vi "basement tank 4.vi"() -> ()   [LabVIEW 2019]
uses:
  <vilib>/NI/Current Value Table/Type Defs/Single Tag.ctl
  <vilib>/NI/Current Value Table/Type Defs/Data Types.ctl
  <vilib>/NI/STM/TCP/Read Meta Data (TCP Ref).vi
  <vilib>/NI/STM/TCP/Get Connection Reference (TCP).vi
  <vilib>/NI/AMC/Read Termination Message.vi
  <vilib>/NI/AMC/Create Single Message.vi
  <vilib>/NI/AMC/Update Message Routing Info.vi
  <vilib>/NI/STM/TCP/Read Meta Data (TCP Clst).vi
  <vilib>/NI/AMC/Globals.vi
  <vilib>/NI/STM/TCP/Write Message (TCP).vi
  <vilib>/NI/AMC/Send Message.vi
  <vilib>/NI/AMC/AMC.lvlib
  <vilib>/NI/STM/NI STM.lvlib
  <vilib>/NI/Current Value Table/Current Value Table.lvlib
panel:
  in  "Specific Gravity":dbl(knob)=1.0 min=1.0 max=1.25 step=0.0025 scale=1.0..1.25
  in  "Pump Speed (%)":dbl(knob) scale=10.0..100.0
  out "Boiler Water Out":dbl(knob) scale=10.0..110.0
  out "Boiler Water In":dbl(knob) scale=10.0..110.0
  out "Tempered Water Out":dbl(knob) scale=10.0..35.0
  out "Tempered Water In":dbl(knob) scale=10.0..35.0
  out "Chilled Water Out":dbl(knob) scale=0.0..25.0
  out "Chilled Water In":dbl(knob) scale=0.0..25.0
  in  "Tab Control":enum32{"Main Pump"}(tab)
  out "Amps":dbl format="%#.2g"
  out "Volts":dbl format="%#.1f"
  out "VFD T":dbl format="%#.2g"
  out "RPM":dbl format="%#.2f"
  out "Fault Code":dbl format="%#.2g"
  out "Freq":dbl format="%#.2g"
  out "Main Pump":bool
  out "Total Added":dbl format="%.2g"
  out "DI Flow (L/min)":dbl(knob) scale=0.0..100.0
  in  "Liters DI to Add":dbl(knob) min=0.0 max=500.0 step=1.0 scale=0.0..500.0
  in  "Add DI Water":bool
  in  "Drain System to Tree":bool
  in  "Enable Main Pump":bool
  out "E Stop":bool
  out "Run Enabled?":bool
  out "Tank":dbl(slide) scale=0.0..1500.0
  in  "Machine":bool
  in  "Basement 4":bool
  in  "Dryer":bool
  in  "Rinse 4":bool
  in  "Rinse 3":bool
  in  "Rinse 2":bool
  in  "Basement 3":bool
  in  "Basement 2":bool
  in  "Basement 1":bool
  in  "Plater 6":bool
  in  "Plater 5":bool
  in  "Plater 4":bool
  in  "Plater 3":bool
  in  "Plater 2":bool
  in  "Plater 1":bool
  in  "Predip":bool
  in  "Rinse 1":bool
  in  "Cleaner":bool
  in  "Etch":bool
  out "status":string
  out "Tnk1Tee":bool
  out "PipeToPump":bool
  # "Module Selection"
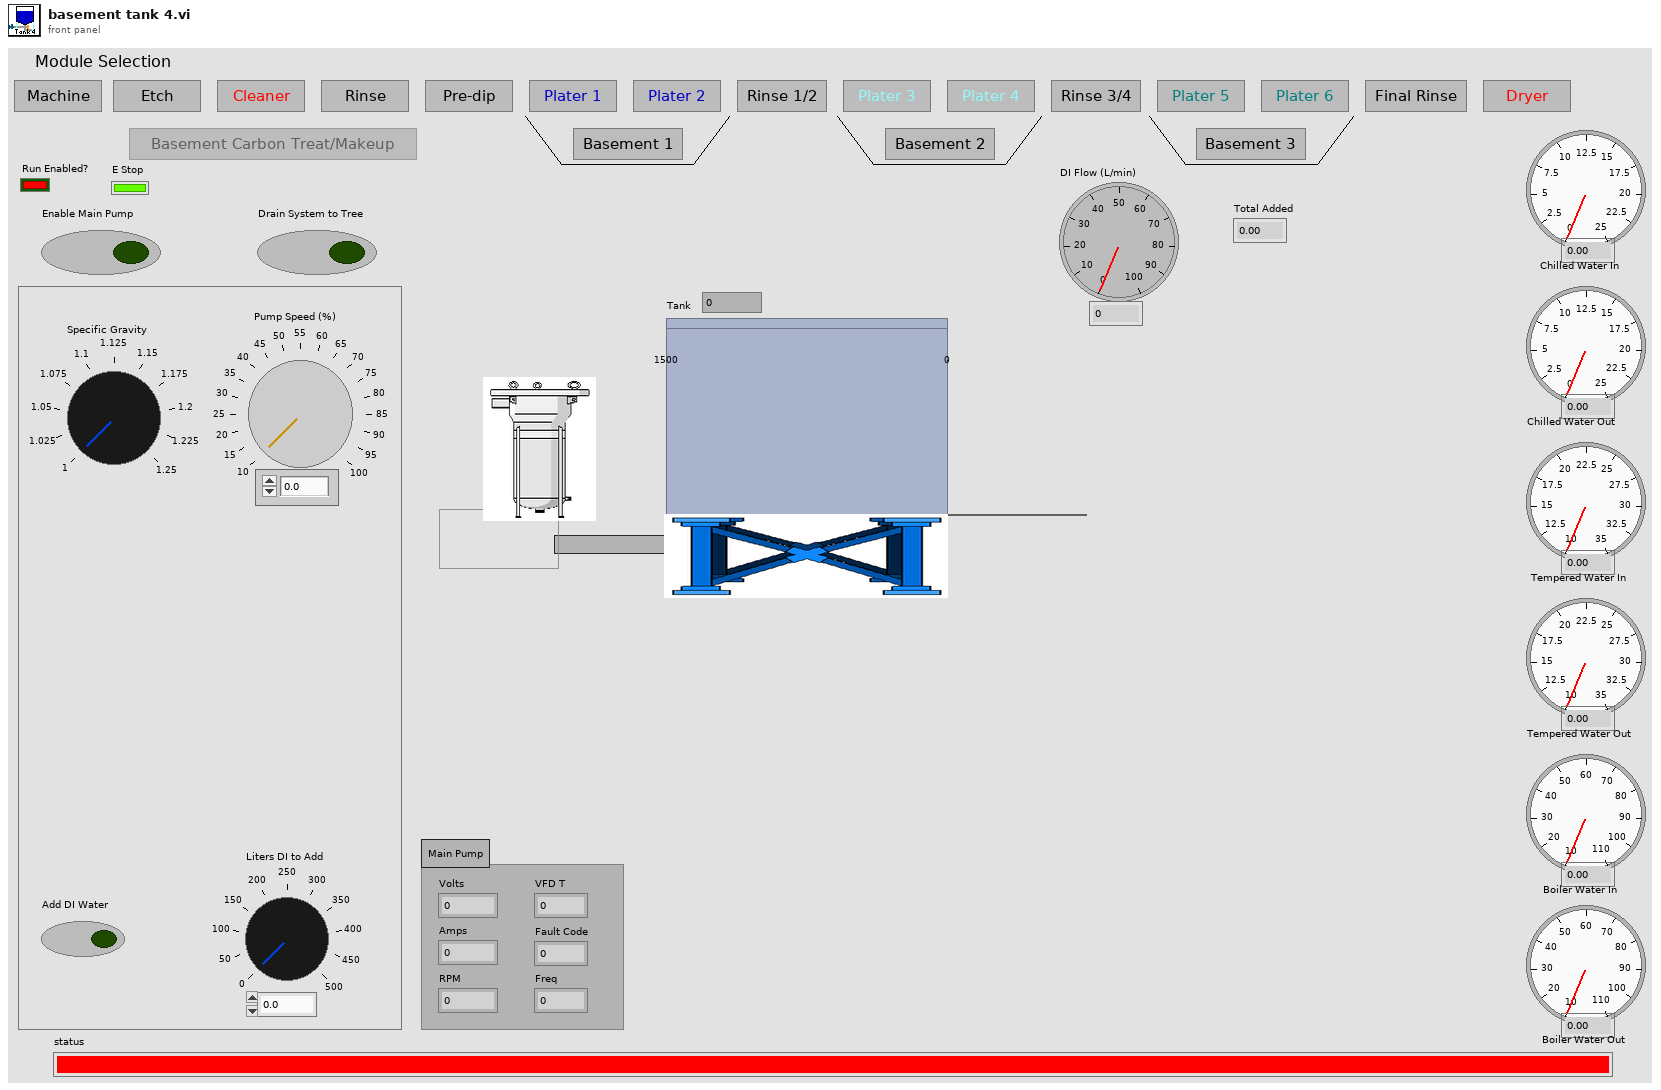
[diagram p1: front panel]
types:
  T1 = typedef "Current Value Table.lvlib/Single Tag.ctl" = cluster{"Data Type":T2, "Name":string, "Value":string, "Description":string}
  T2 = typedef "Current Value Table.lvlib/Data Types.ctl" = enum16{"Double", "Single", "I64", "I32", "I16", "I8", "U64", "U32", "U16", "U8", "String", "Boolean", "Array of U8", "Array of U16", "Array of U32", "Array of U64", "Array of I64", "Array of I32", "Array of I16", "Array of I8", "Array of Double", "Array of Single", "Array of Boolean", "Array of String"}
  T3 = typedef "NI STM.lvlib/TCP Connection Info.ctl" = cluster{"connection ID":refnum<k5>, "meta data":T4[]}
  T4 = typedef "NI STM.lvlib/MetaDataElement.ctl" = string
  T5 = typedef "AMC.lvlib/Message Queue.ctl" = refnum<queue>
  T6 = enum8{"Enabled", "Disabled", "Disabled and Grayed Out"}
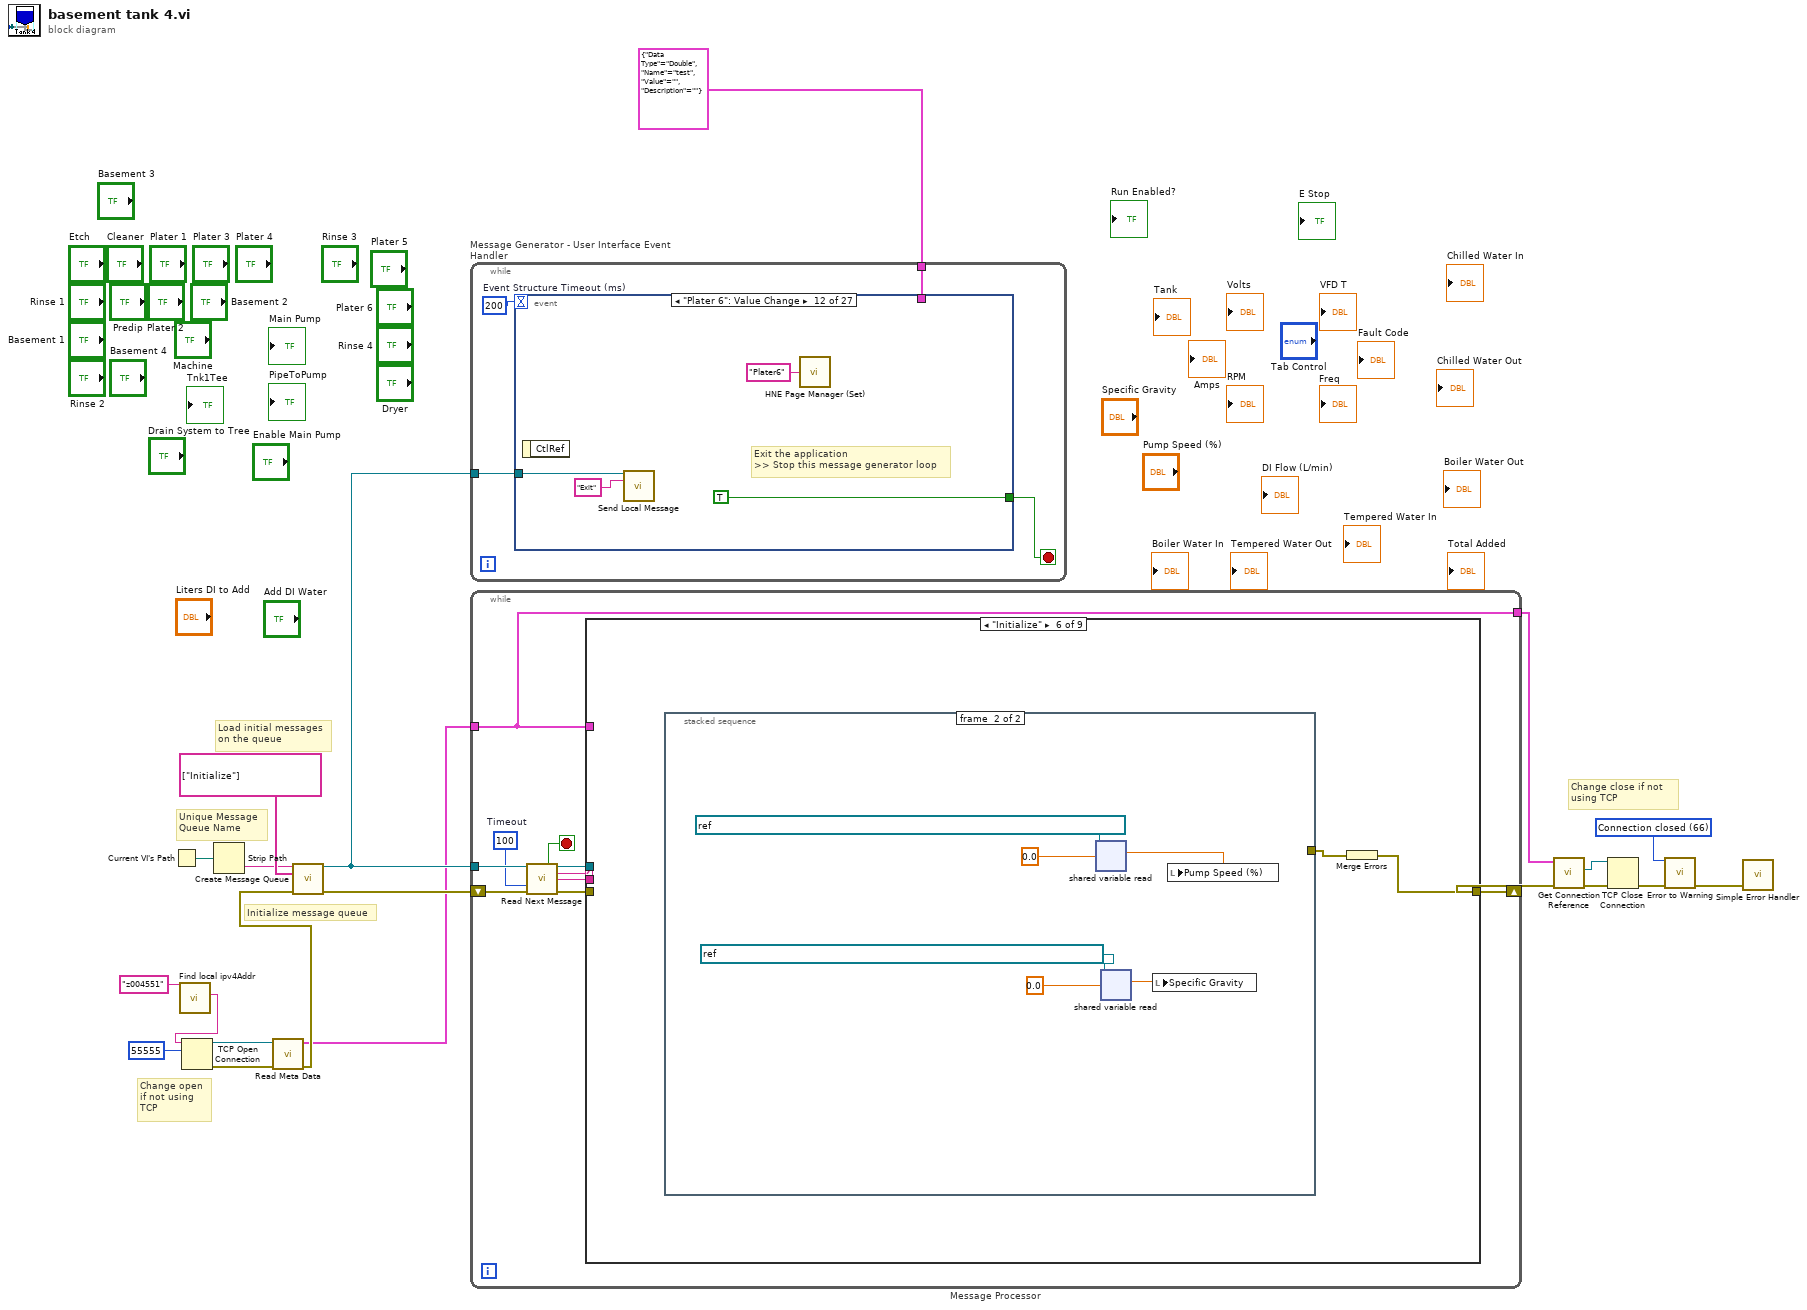
[diagram p0: block diagram]
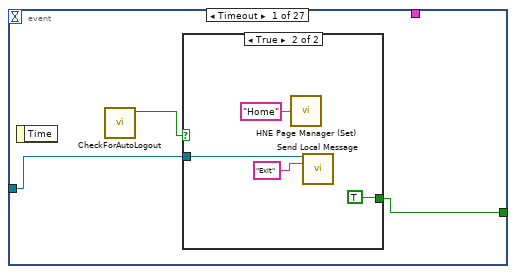
[diagram p2: hidden frame]
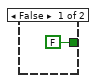
[diagram p3: hidden frame]
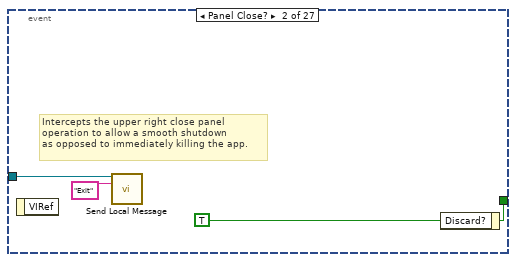
[diagram p4: hidden frame]
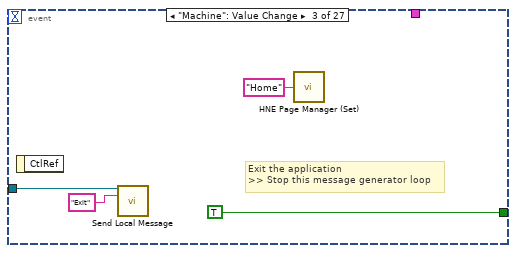
[diagram p5: hidden frame]
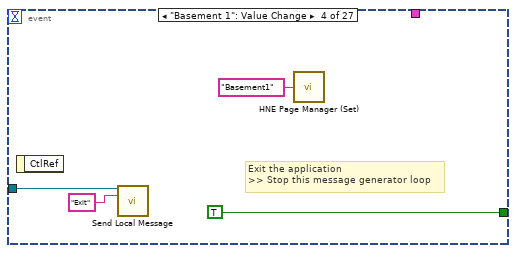
[diagram p6: hidden frame]
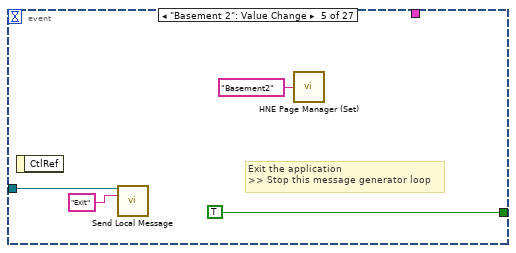
[diagram p7: hidden frame]
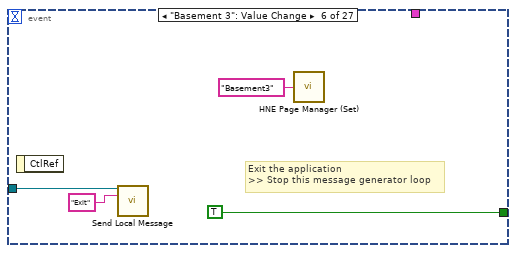
[diagram p8: hidden frame]
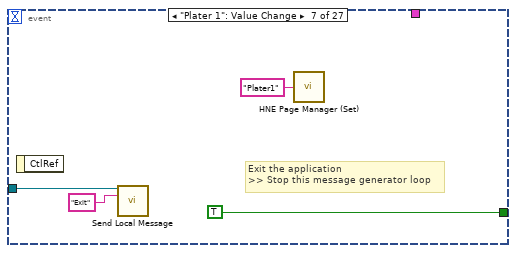
[diagram p9: hidden frame]
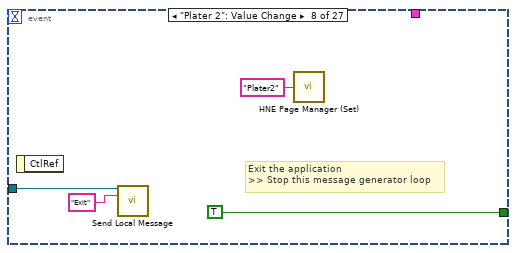
[diagram p10: hidden frame]
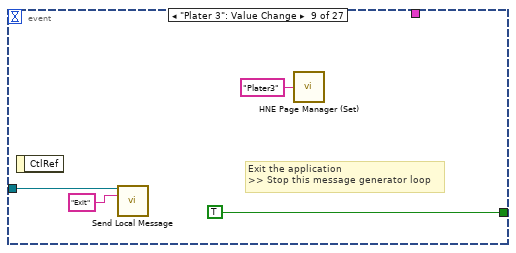
[diagram p11: hidden frame]
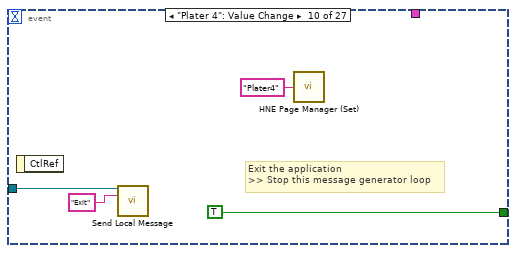
[diagram p12: hidden frame]
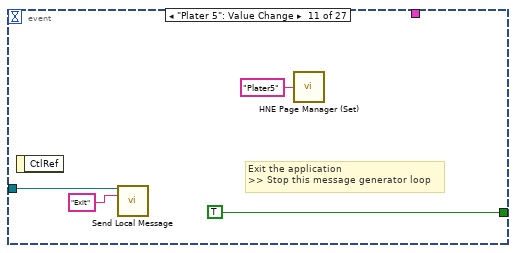
[diagram p13: hidden frame]
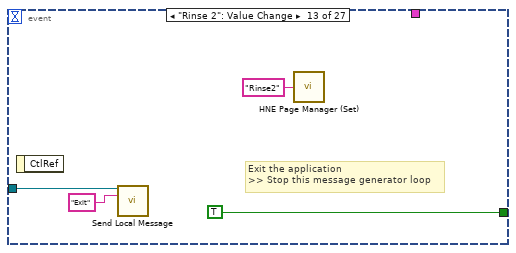
[diagram p14: hidden frame]
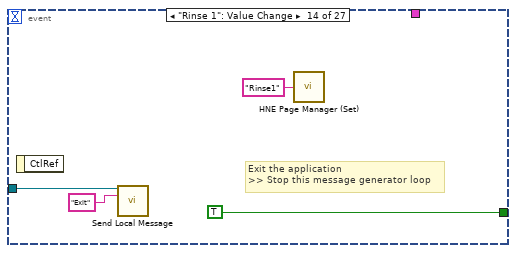
[diagram p15: hidden frame]
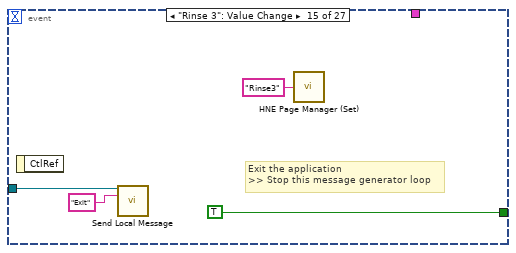
[diagram p16: hidden frame]
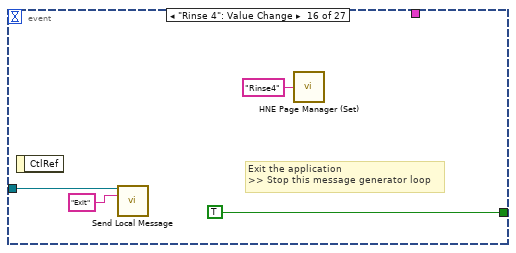
[diagram p17: hidden frame]
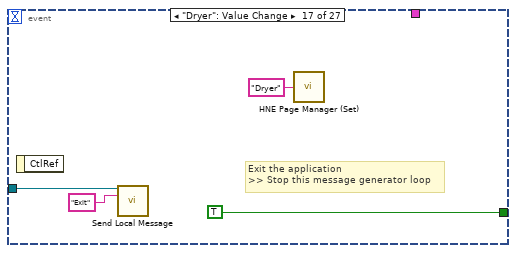
[diagram p18: hidden frame]
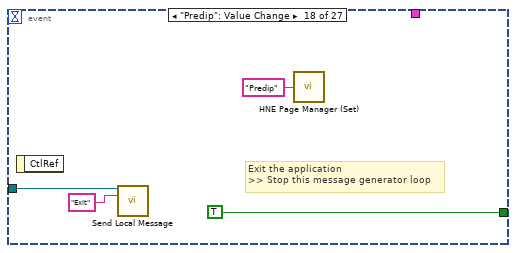
[diagram p19: hidden frame]
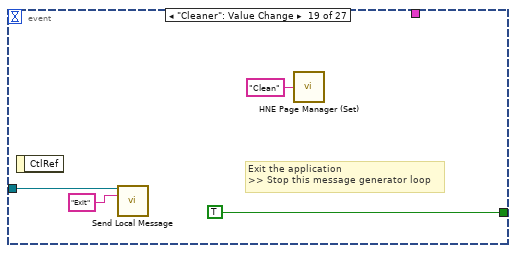
[diagram p20: hidden frame]
diagram:
  w9 = 66 items=["No Error", "Argument Error", "Memory Full", "Out of Zone", "End of File", "File Already Open", "Generic File IO Error", "File Not Found", "File Permission Error", "Disk Full", "Duplicate Path", "Too Many Files Open", "Not Enabled", "Resource File Not Found", "Cannot Add Resource", "Resource Not Found", "Image Not Found", "Image Memory Error", "Pen Does Not Exist", "Config Bad Type", "Config Token Not Found", "Config Parse Error", "Config Memory Error", "Bad External Code Format", "Bad External Code Offset", "External Code Not Present", "Null Window", "Destroy Window Mixup", "Null Menu", "Print Aborted", "Bad Print Record", "Print Driver Error", "Windows Error During Print", "Memory Error During Print", "Print Dialog Error", "Generic Print Error", "Invalid Device Refnum", "Device Not Found", "Device Parameter Error", "Device Unit Error", "Can't Open Device", "Device Call Aborted", "Generic Error", "Cancelled By User", "Object ID Too Low", "Object ID Too High", "Object Not In Heap", "Unknown Heap", "Bad DefProc ID", "DefProc Not In Table", "Message Out Of Range", "Null Method", "Unknown Message", "Manager Call Not Supported", "Bad address", "Connection In progress", "Connection timed out", "Connection is already in progress", "Network attribute not supported", "Network error", "Address in use", "System out of memory", "Connection aborted", "Connection refused", "Connection is not connected", "Connection is already connected", "Connection closed", "Initialize error (interapplication manager)", "Bad occurrence", "Wait on unbound occurrence handler", "Occurrence queue overflow", "Bad path", "Semaphore not signaled", "Unrecognized type (interapplication manager)"] ("1st Error to Convert")
  # "Change close if not using TCP"
  # "Change open if not using TCP"
  # "Initialize message queue"
  # "Unique Message\nQueue Name"
  # "Load initial messages\non the queue"
  n1 = Current VI's Path() -> (path=w16:path)
  n2 = call "Find local ipv4Addr.vi"("MachineToFind"="z004551" ("Target IP Address")) -> ("name"=w1:string)  [unwired: 9 in, 1 out]
  n3 = TCP Open Connection(address=w1, remote port or service name=u16 55555 ("remote port")) -> (connection ID=w14:refnum<k5>, error out=w13:errorcluster)  [unwired: 1 in, 2 out]
  n4 = Strip Path(path=w16) -> (name=w19:string)  [unwired: 1 out]
  n5 = call-poly <vilib>:"Read Meta Data.vi"("error in"=w13, "connection ID"=w14) -> ("error out"=w12:errorcluster, "connection info out"=w11:T3)  [unwired: 7 in, 1 out]
  n6 = call <vilib>:"Create Message Queue.vi"("message queue name"=w19, "initial message names"=string[] ["Initialize"], "error in"=w12) -> ("message queue out"=w18:T5, "error out"=w17:errorcluster)  [unwired: 11 in]
  n7 = while "Message Generator - User Interface Event Handler" {
    tunnel: w18 -> [w22]
    tunnel: T1 {"Data Type"=enum."Double", "Name"="test", "Value"="", "Description"=""} ("Tag") -> [w21]
    stop <- w23 stop-if-true
    w24 = 200  # Event Structure Timeout (ms)
    n8 = event shown="[11] \"Plater 6\": Value Change" {
      selector: _ -> [_ _ _ _ _ _ _ _ _ _ _ _ _ _ _ _ _ _ _ _ _ _ _ _ _ _ _]
      dyn-events: _ -> [_ _ _ _ _ _ _ _ _ _ _ _ _ _ _ _ _ _ _ _ _ _ _ _ _ _ _]
      timeout: w24 -> [_ _ _ _ _ _ _ _ _ _ _ _ _ _ _ _ _ _ _ _ _ _ _ _ _ _ _]
      tunnel: [w25 w35 TRUE ("Discard?") TRUE ("Discard?") TRUE ("Discard?") TRUE ("Discard?") TRUE ("Discard?") TRUE ("Discard?") TRUE ("Discard?") TRUE ("Discard?") TRUE ("Discard?") TRUE ("Discard?") TRUE ("Discard?") TRUE ("Discard?") TRUE ("Discard?") TRUE ("Discard?") TRUE ("Discard?") TRUE ("Discard?") TRUE ("Discard?") TRUE ("Discard?") _ _ _ _ _ _ _] -> w23
      tunnel: w22 -> [w26 w33 w37 w41 w45 w49 w53 w57 w61 w65 w69 w73 w77 w81 w85 w89 w93 w97 w101 w105 w108 w119 w129 w139 w148 w157 w166]
      tunnel: w21 -> [_ _ _ _ _ _ _ _ _ _ _ _ _ _ _ _ _ _ _ _ _ w113 w123 w133 w144 w153 w162]
      event Timeout {
        n9 = event-data() -> ()  [unwired: 2 out]
        n10 = call "CheckForAutoLogout.vi"() -> ("Boolean"=w27:bool)  [unwired: 11 in]
        n11 = case shown="True" w27 {
          tunnel: [FALSE ("Discard?") TRUE ("Discard?")] -> w25
          tunnel: w26 -> [_ w29]
          frame False {
          }
          frame True {
            n12 = call <userlib>:"HNE Page Manager (Set).vi"("Next Page"="Home") -> ()  [unwired: 4 in, 1 out]
            n13 = call <vilib>:"Send Local Message.vi"("message queue in"=w29, "message name"="Exit") -> ()  [unwired: 11 in, 3 out]
          }
        }
      }
      event Panel Close? {
        w35 = TRUE ("Discard?")
        # "Intercepts the upper right close panel\noperation to allow a smooth shutdown\nas opposed to immediately killing the app."
        n14 = event-data() -> ()  [unwired: 2 out]
        n15 = call <vilib>:"Send Local Message.vi"("message queue in"=w33, "message name"="Exit") -> ()  [unwired: 11 in, 3 out]
        n16 = event-data("Discard?"=w35) -> ()  [unwired: 1 in, 1 out]
      }
      event "Machine": Value Change {
        # "Exit the application\n>> Stop this message generator loop"
        n17 = event-data() -> ()  [unwired: 2 out]
        n18 = call <vilib>:"Send Local Message.vi"("message queue in"=w37, "message name"="Exit") -> ()  [unwired: 11 in, 3 out]
        n19 = call <userlib>:"HNE Page Manager (Set).vi"("Next Page"="Home") -> ()  [unwired: 4 in, 1 out]
      }
      event "Basement 1": Value Change {
        # "Exit the application\n>> Stop this message generator loop"
        n20 = event-data() -> ()  [unwired: 2 out]
        n21 = call <vilib>:"Send Local Message.vi"("message queue in"=w41, "message name"="Exit") -> ()  [unwired: 11 in, 3 out]
        n22 = call <userlib>:"HNE Page Manager (Set).vi"("Next Page"="Basement1") -> ()  [unwired: 4 in, 1 out]
      }
      event "Basement 2": Value Change {
        # "Exit the application\n>> Stop this message generator loop"
        n23 = event-data() -> ()  [unwired: 2 out]
        n24 = call <vilib>:"Send Local Message.vi"("message queue in"=w45, "message name"="Exit") -> ()  [unwired: 11 in, 3 out]
        n25 = call <userlib>:"HNE Page Manager (Set).vi"("Next Page"="Basement2") -> ()  [unwired: 4 in, 1 out]
      }
      event "Basement 3": Value Change {
        # "Exit the application\n>> Stop this message generator loop"
        n26 = event-data() -> ()  [unwired: 2 out]
        n27 = call <vilib>:"Send Local Message.vi"("message queue in"=w49, "message name"="Exit") -> ()  [unwired: 11 in, 3 out]
        n28 = call <userlib>:"HNE Page Manager (Set).vi"("Next Page"="Basement3") -> ()  [unwired: 4 in, 1 out]
      }
      event "Plater 1": Value Change {
        # "Exit the application\n>> Stop this message generator loop"
        n29 = event-data() -> ()  [unwired: 2 out]
        n30 = call <vilib>:"Send Local Message.vi"("message queue in"=w53, "message name"="Exit") -> ()  [unwired: 11 in, 3 out]
        n31 = call <userlib>:"HNE Page Manager (Set).vi"("Next Page"="Plater1") -> ()  [unwired: 4 in, 1 out]
      }
      event "Plater 2": Value Change {
        # "Exit the application\n>> Stop this message generator loop"
        n32 = event-data() -> ()  [unwired: 2 out]
        n33 = call <vilib>:"Send Local Message.vi"("message queue in"=w57, "message name"="Exit") -> ()  [unwired: 11 in, 3 out]
        n34 = call <userlib>:"HNE Page Manager (Set).vi"("Next Page"="Plater2") -> ()  [unwired: 4 in, 1 out]
      }
      event "Plater 3": Value Change {
        # "Exit the application\n>> Stop this message generator loop"
        n35 = event-data() -> ()  [unwired: 2 out]
        n36 = call <vilib>:"Send Local Message.vi"("message queue in"=w61, "message name"="Exit") -> ()  [unwired: 11 in, 3 out]
        n37 = call <userlib>:"HNE Page Manager (Set).vi"("Next Page"="Plater3") -> ()  [unwired: 4 in, 1 out]
      }
      event "Plater 4": Value Change {
        # "Exit the application\n>> Stop this message generator loop"
        n38 = event-data() -> ()  [unwired: 2 out]
        n39 = call <vilib>:"Send Local Message.vi"("message queue in"=w65, "message name"="Exit") -> ()  [unwired: 11 in, 3 out]
        n40 = call <userlib>:"HNE Page Manager (Set).vi"("Next Page"="Plater4") -> ()  [unwired: 4 in, 1 out]
      }
      event "Plater 5": Value Change {
        # "Exit the application\n>> Stop this message generator loop"
        n41 = event-data() -> ()  [unwired: 2 out]
        n42 = call <vilib>:"Send Local Message.vi"("message queue in"=w69, "message name"="Exit") -> ()  [unwired: 11 in, 3 out]
        n43 = call <userlib>:"HNE Page Manager (Set).vi"("Next Page"="Plater5") -> ()  [unwired: 4 in, 1 out]
      }
      event "Plater 6": Value Change {
        # "Exit the application\n>> Stop this message generator loop"
        n44 = event-data() -> ()  [unwired: 2 out]
        n45 = call <vilib>:"Send Local Message.vi"("message queue in"=w73, "message name"="Exit") -> ()  [unwired: 11 in, 3 out]
        n46 = call <userlib>:"HNE Page Manager (Set).vi"("Next Page"="Plater6") -> ()  [unwired: 4 in, 1 out]
      }
      event "Rinse 2": Value Change {
        # "Exit the application\n>> Stop this message generator loop"
        n47 = event-data() -> ()  [unwired: 2 out]
        n48 = call <vilib>:"Send Local Message.vi"("message queue in"=w77, "message name"="Exit") -> ()  [unwired: 11 in, 3 out]
        n49 = call <userlib>:"HNE Page Manager (Set).vi"("Next Page"="Rinse2") -> ()  [unwired: 4 in, 1 out]
      }
      event "Rinse 1": Value Change {
        # "Exit the application\n>> Stop this message generator loop"
        n50 = event-data() -> ()  [unwired: 2 out]
        n51 = call <vilib>:"Send Local Message.vi"("message queue in"=w81, "message name"="Exit") -> ()  [unwired: 11 in, 3 out]
        n52 = call <userlib>:"HNE Page Manager (Set).vi"("Next Page"="Rinse1") -> ()  [unwired: 4 in, 1 out]
      }
      event "Rinse 3": Value Change {
        # "Exit the application\n>> Stop this message generator loop"
        n53 = event-data() -> ()  [unwired: 2 out]
        n54 = call <vilib>:"Send Local Message.vi"("message queue in"=w85, "message name"="Exit") -> ()  [unwired: 11 in, 3 out]
        n55 = call <userlib>:"HNE Page Manager (Set).vi"("Next Page"="Rinse3") -> ()  [unwired: 4 in, 1 out]
      }
      event "Rinse 4": Value Change {
        # "Exit the application\n>> Stop this message generator loop"
        n56 = event-data() -> ()  [unwired: 2 out]
        n57 = call <vilib>:"Send Local Message.vi"("message queue in"=w89, "message name"="Exit") -> ()  [unwired: 11 in, 3 out]
        n58 = call <userlib>:"HNE Page Manager (Set).vi"("Next Page"="Rinse4") -> ()  [unwired: 4 in, 1 out]
      }
      event "Dryer": Value Change {
        # "Exit the application\n>> Stop this message generator loop"
        n59 = event-data() -> ()  [unwired: 2 out]
        n60 = call <vilib>:"Send Local Message.vi"("message queue in"=w93, "message name"="Exit") -> ()  [unwired: 11 in, 3 out]
        n61 = call <userlib>:"HNE Page Manager (Set).vi"("Next Page"="Dryer") -> ()  [unwired: 4 in, 1 out]
      }
      event "Predip": Value Change {
        # "Exit the application\n>> Stop this message generator loop"
        n62 = event-data() -> ()  [unwired: 2 out]
        n63 = call <vilib>:"Send Local Message.vi"("message queue in"=w97, "message name"="Exit") -> ()  [unwired: 11 in, 3 out]
        n64 = call <userlib>:"HNE Page Manager (Set).vi"("Next Page"="Predip") -> ()  [unwired: 4 in, 1 out]
      }
      event "Cleaner": Value Change {
        # "Exit the application\n>> Stop this message generator loop"
        n65 = event-data() -> ()  [unwired: 2 out]
        n66 = call <vilib>:"Send Local Message.vi"("message queue in"=w101, "message name"="Exit") -> ()  [unwired: 11 in, 3 out]
        n67 = call <userlib>:"HNE Page Manager (Set).vi"("Next Page"="Clean") -> ()  [unwired: 4 in, 1 out]
      }
      event "Etch": Value Change {
        # "Exit the application\n>> Stop this message generator loop"
        n68 = event-data() -> ()  [unwired: 2 out]
        n69 = call <vilib>:"Send Local Message.vi"("message queue in"=w105, "message name"="Exit") -> ()  [unwired: 11 in, 3 out]
        n70 = call <userlib>:"HNE Page Manager (Set).vi"("Next Page"="Etch") -> ()  [unwired: 4 in, 1 out]
      }
      event Menu Selection (User) {
        # "Add run-time menu items to the message\nqueue. The message handler case names must match the menu ItemTag names."
        n71 = event-data() -> ("ItemTag"=w109:string)  [unwired: 1 out]
        n72 = call <vilib>:"Send Local Message.vi"("message queue in"=w108, "message name"=w109) -> ()  [unwired: 11 in, 3 out]
      }
      event "Enable Main Pump": Value Change {
        n73 = event-data() -> ("NewVal"=w112:bool)  [unwired: 1 out]
        n74 = Boolean To (0,1)(Boolean=w112) -> (0, 1=w118:i16)
        n75 = Number To Decimal String(number=w118) -> (decimal integer string=w117:string)  [unwired: 1 in]
        n76 = Bundle By Name(cluster=w113, "Data Type"=Data_Types."Boolean", "Name"="HMI_Enable_BTnk4_Pump", "Value"=w117) -> (w116:T1)
        n77 = Flatten To String(anything=w116) -> (data string=w110:string)  [unwired: 3 in, 2 out]
        n78 = call <vilib>:"Send Local Message.vi"("message queue in"=w119, "message name"="Write_Tag", "message value"=w110) -> ()  [unwired: 10 in, 3 out]
      }
      event "Drain System to Tree": Value Change {
        n79 = event-data() -> ("NewVal"=w122:bool)  [unwired: 1 out]
        n80 = Boolean To (0,1)(Boolean=w122) -> (0, 1=w128:i16)
        n81 = Number To Decimal String(number=w128) -> (decimal integer string=w127:string)  [unwired: 1 in]
        n82 = Bundle By Name(cluster=w123, "Data Type"=Data_Types."Boolean", "Name"="HMI_Drain_BTank4", "Value"=w127) -> (w126:T1)
        n83 = Flatten To String(anything=w126) -> (data string=w120:string)  [unwired: 3 in, 2 out]
        n84 = call <vilib>:"Send Local Message.vi"("message queue in"=w129, "message name"="Write_Tag", "message value"=w120) -> ()  [unwired: 10 in, 3 out]
      }
      event "Add DI Water": Value Change {
        n85 = event-data() -> ("NewVal"=w132:bool)  [unwired: 1 out]
        n86 = Boolean To (0,1)(Boolean=w132) -> (0, 1=w138:i16)
        n87 = Number To Decimal String(number=w138) -> (decimal integer string=w137:string)  [unwired: 1 in]
        n88 = Bundle By Name(cluster=w133, "Data Type"=Data_Types."Boolean", "Name"="HMI_BAS_Proc4_AddDIVolume", "Value"=w137) -> (w136:T1)
        n89 = Flatten To String(anything=w136) -> (data string=w130:string)  [unwired: 3 in, 2 out]
        n90 = call <vilib>:"Send Local Message.vi"("message queue in"=w139, "message name"="Write_Tag", "message value"=w130) -> ()  [unwired: 10 in, 3 out]
      }
      event "Liters DI to Add": Value Change {
        n91 = event-data() -> ("NewVal"=w141:dbl)  [unwired: 1 out]
        n92 = Number To Fractional String(number=w141) -> (F-format string=w140:string)  [unwired: 3 in]
        n93 = Bundle By Name(cluster=w144, "Data Type"=Data_Types."Double", "Name"="HMI_BAS_Proc4_DI_Setpnt", "Value"=w140) -> (w147:T1)
        n94 = Flatten To String(anything=w147) -> (data string=w142:string)  [unwired: 3 in, 2 out]
        n95 = call <vilib>:"Send Local Message.vi"("message queue in"=w148, "message name"="Write_Tag", "message value"=w142) -> ()  [unwired: 10 in, 3 out]
      }
      event "Pump Speed (%)": Value Change {
        n96 = event-data() -> ("NewVal"=w150:dbl)  [unwired: 1 out]
        n97 = Number To Fractional String(number=w150) -> (F-format string=w149:string)  [unwired: 3 in]
        n98 = Bundle By Name(cluster=w153, "Data Type"=Data_Types."Double", "Name"="HMI_BAS_Tnk4RecircPmpPcnt", "Value"=w149) -> (w156:T1)
        n99 = Flatten To String(anything=w156) -> (data string=w151:string)  [unwired: 3 in, 2 out]
        n100 = call <vilib>:"Send Local Message.vi"("message queue in"=w157, "message name"="Write_Tag", "message value"=w151) -> ()  [unwired: 10 in, 3 out]
      }
      event "Specific Gravity": Value Change {
        n101 = event-data() -> ("NewVal"=w159:dbl)  [unwired: 1 out]
        n102 = Number To Fractional String(number=w159) -> (F-format string=w158:string)  [unwired: 3 in]
        n103 = Bundle By Name(cluster=w162, "Data Type"=Data_Types."Double", "Name"="HMI_BAS_Proc4_Tank_SG", "Value"=w158) -> (w165:T1)
        n104 = Flatten To String(anything=w165) -> (data string=w160:string)  [unwired: 3 in, 2 out]
        n105 = call <vilib>:"Send Local Message.vi"("message queue in"=w166, "message name"="Write_Tag", "message value"=w160) -> ()  [unwired: 10 in, 3 out]
      }
    }
  }
  n106 = while "Message Processor" {
    shift-left: w17 -> [w172]
    shift-right: [w176] -> w4
    tunnel: w18 -> [w173]
    tunnel: w11 -> [w167]
    tunnel: [w167] -> w5
    stop <- w175 stop-if-true
    w168 = 100  # Timeout
    n107 = call <vilib>:"Read Next Message.vi"("message queue in"=w173, "timeout (1 ms)"=w168, "error in"=w172) -> ("exit process?"=w175:bool, "message queue out"=w174:T5, "message name"=w170:string, "message value"=w169:string, "error out"=w171:errorcluster)  [unwired: 5 in, 3 out]
    n108 = case shown="\"Initialize\"" w170 {
      selector: w170 -> [_ _ w206 _ _ _ _ _ _]
      tunnel: w174 -> [_ _ _ _ _ _ w235 _ _]
      tunnel: w171 -> [w177 _ w207 w208 w210 _ w236 w238 w240]
      tunnel: [w177 w179 w207 errorcluster {"status"=FALSE, "code"=0, "source"=""} ("error out") w210 w211 w234 w238 w239] -> w176
      tunnel: w169 -> [_ _ _ _ _ _ _ _ w241]
      tunnel: w167 -> [_ _ _ _ _ _ _ _ w243]
      frame "---------- Framework Operations ----------" {
        # "Dummy case to add a seperator in the Case Structure menu"
      }
      frame "", "Idle" {
        n109 = stacked-sequence {
          tunnel: [w187] -> w178
          frame #0 {
            n110 = shared-variable-read(refnum<k21> "ni.var.psp://z004551/CDL0100 ReadWriteTags/HMI_Drain_BTank4" ("shared variable refnum in"), FALSE) -> (w181:errorcluster, w184:bool)  [unwired: 1 in, 2 out]
            n111 = shared-variable-read(refnum<k21> "ni.var.psp://z004551/CDL0100 ReadWriteTags/HMI_BAS_Proc4_AddDIVolume" ("shared variable refnum in"), FALSE) -> (w188:errorcluster, w191:bool)  [unwired: 1 in, 2 out]
            n112 = shared-variable-read(refnum<k21> "ni.var.psp://z004551/CDL0100 ReadWriteTags/HMI_Enable_BTnk4_Pump" ("shared variable refnum in"), FALSE) -> (w189:errorcluster, w196:bool)  [unwired: 1 in, 2 out]
            n113 = call <userlib>:"Boolean Trigger__ogtk.vi"("Boolean Input"=w191) -> ("Falling Edge"=w190:bool)  [unwired: 1 in, 1 out]
            n114 = case shown="True" w184 {
              tunnel: [T6."Enabled" ("Disabled") T6."Disabled and Grayed Out" ("Disabled")] -> w183
              frame False {
              }
              frame True {
              }
            }
            n115 = case shown="True" w196 {
              tunnel: [T6."Enabled" ("Disabled") T6."Disabled and Grayed Out" ("Disabled")] -> w195
              frame False {
              }
              frame True {
              }
            }
            n116 = control-ref of="Drain System to Tree"() -> (w194:refnum<vi>)
            n117 = case shown="True" w190 {
              frame False {
              }
              frame True {
                n118 = local write "Add DI Water"(FALSE) -> ()
              }
            }
            n119 = control-ref of="Enable Main Pump"() -> (w182:refnum<vi>)
            n120 = property class="Bool (strict)"(reference=w194, "DisabledEnum"=w195) -> ()  [unwired: 1 in, 2 out]
            n121 = property class="Bool (strict)"(reference=w182, "DisabledEnum"=w183) -> ()  [unwired: 1 in, 2 out]
            n122 = Merge Errors(w189, w188, w181) -> (w187:errorcluster)
          }
        }
        n123 = control-ref of="status"() -> (w180:refnum<vi>)
        n124 = call <userlib>:"TAE Format Alarm Ticker.vi"("Alarm Ticker Ref"=w180) -> ()  [unwired: 15 in]
        n125 = Merge Errors(w178) -> (w179:errorcluster)
      }
      frame "Missing Message Handler", Default {
        # "Call this case if a message is received that is not handled \nby any other case. Typically this is a programming error\nas a result of a typo or unhandled message/missing message handler."
        n126 = Format Into String(format string="DevError: Missing message handler for '%s\" message." ("message"), w206) -> (resulting string=w204:string)  [unwired: 2 in, 1 out]
        n127 = One Button Dialog(message=w204) -> ()  [unwired: 2 out]
      }
      frame "Error" {
        # "General Error Case - this case is called if an error is passed using the error cluster below. Typically most new errors should be handed in each individual case and not passed in the rror cluster. If necessary a custom error handler case should be added and called from other cases."
        n128 = call <vilib>:"Simple Error Handler.vi"("error in (no error)"=w208) -> ()  [unwired: 1 in, 8 out]
      }
      frame "---------- Generic Operations ----------" {
        # "Dummy case to add a seperator in the Case Structure menu"
      }
      frame "Initialize" {
        n129 = stacked-sequence {
          tunnel: [w219 _] -> w212
          frame #0 {
            n130 = shared-variable-read(refnum<k21> "ni.var.psp://z004551/CDL0100 ReadWriteTags/HMI_Drain_BTank4" ("shared variable refnum in"), FALSE) -> (w220:errorcluster, w222:bool)  [unwired: 1 in, 2 out]
            n131 = shared-variable-read(refnum<k21> "ni.var.psp://z004551/CDL0100 ReadWriteTags/HMI_BAS_Proc4_AddDIVolume" ("shared variable refnum in"), FALSE) -> (w213:bool)  [unwired: 1 in, 3 out]
            n132 = shared-variable-read(refnum<k21> "ni.var.psp://z004551/CDL0100 ReadWriteTags/HMI_Enable_BTnk4_Pump" ("shared variable refnum in"), FALSE) -> (w221:errorcluster, w225:bool)  [unwired: 1 in, 2 out]
            n133 = shared-variable-read(refnum<k21> "ni.var.psp://z004551/CDL0100 ReadWriteTags/HMI_BAS_Proc4_DI_Setpnt" ("shared variable refnum in"), 0.0) -> (w214:dbl)  [unwired: 1 in, 3 out]
            n134 = local write "Drain System to Tree"(w222) -> ()
            n135 = local write "Add DI Water"(w213) -> ()
            n136 = local write "Enable Main Pump"(w225) -> ()
            n137 = local write "Liters DI to Add"(w214) -> ()
            n138 = Merge Errors(w221, w220) -> (w219:errorcluster)
          }
          frame #1 {
            n139 = shared-variable-read(refnum<k21> "ni.var.psp://z004551/CDL0100 ReadWriteTags/HMI_BAS_Tnk4RecircPmpPcnt" ("shared variable refnum in"), 0.0) -> (w231:dbl)  [unwired: 1 in, 3 out]
            n140 = shared-variable-read(refnum<k21> "ni.var.psp://z004551/CDL0100 ReadWriteTags/HMI_BAS_Proc4_Tank_SG" ("shared variable refnum in"), 0.0) -> (w228:dbl)  [unwired: 1 in, 3 out]
            n141 = local write "Specific Gravity"(w228) -> ()
            n142 = local write "Pump Speed (%)"(w231) -> ()
          }
        }
        n143 = Merge Errors(w212) -> (w211:errorcluster)
      }
      frame "Exit" {
        # "Destroy message queue >> this will halt the UI event handler loop"
        # "Stop the VI\n>> Perform any cleanup tasks in this message case.\n>> Clear display before closing."
        n144 = call <vilib>:"Destroy Message Queue.vi"("message queue in"=w235, "error in"=w236) -> ("error out"=w234:errorcluster)  [unwired: 11 in, 2 out]
        n145 = local write "status"("" ("Status")) -> ()
      }
      frame "---------- Application Operations ----------" {
        # "Dummy case to add a seperator in the Case Structure menu"
      }
      frame "Write_Tag" {
        n146 = call-poly <vilib>:"Write Message.vi"("error in"=w240, "data"=w241, "name"="WriteTag", "connection info in"=w243) -> ("error out"=w239:errorcluster)  [unwired: 6 in, 1 out]
      }
    }
  }
  n147 = call-poly <vilib>:"Get Connection Reference.vi"("error in"=w4, "connection info in"=w5) -> ("error out"=w8:errorcluster, "connection ID out"=w7:refnum<k5>)  [unwired: 8 out]
  n148 = TCP Close Connection(connection ID=w7, error in (no error)=w8) -> (error out=w10:errorcluster)  [unwired: 2 out]
  n149 = call <vilib>:"Error to Warning.vi"("1st Error to Convert"=w9, "error in"=w10) -> ("warning out"=w6:errorcluster)  [unwired: 3 in, 10 out]
  n150 = call <vilib>:"Simple Error Handler.vi"("error in (no error)"=w6) -> ()  [unwired: 4 in, 5 out]
